vi "Queue_LV2.vi"(0 "name":string, 2 "Queue Operations":T1(ring), 5 "States[]":string[](array[string]), 7 "State":string, 11 "error in":errorcluster) -> (4 "DQ State":string, 15 "error out":errorcluster)   [LabVIEW 2020, in "Airplane CLD1.lvlib"]
uses:
  Airplane CLD1.lvlib
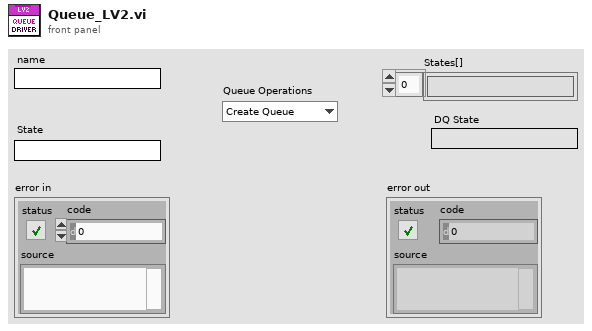
[diagram p1: front panel]
types:
  T1 = enum16{"Create Queue", "Enqueue element", "Enqueue N elements", "Dequeue", "Enstack 1 element", "Flush Queue", "Close Queue"}
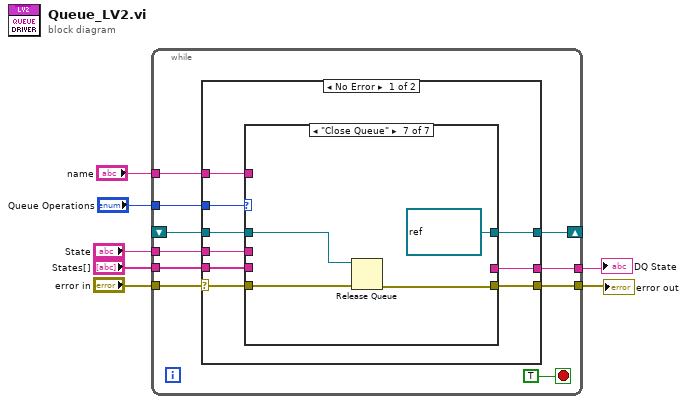
[diagram p0: block diagram]
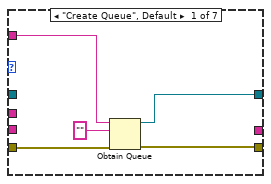
[diagram p2: hidden frame]
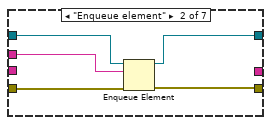
[diagram p3: hidden frame]
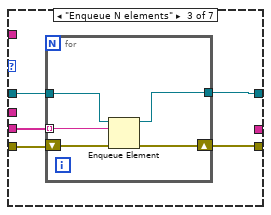
[diagram p4: hidden frame]
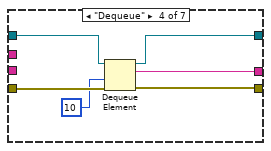
[diagram p5: hidden frame]
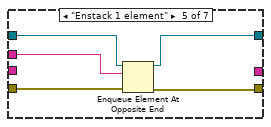
[diagram p6: hidden frame]
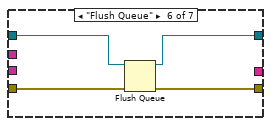
[diagram p7: hidden frame]
diagram:
  n1 = while {
    tunnel: "error in" -> [w17]
    tunnel: [w16] -> w6
    tunnel: "Queue Operations" -> [w15]
    tunnel: "name" -> [w14]
    shift-right: [w12] -> _
    shift-left: _ -> [w13]
    tunnel: "States[]" -> [w11]
    tunnel: "State" -> [w10]
    tunnel: [w9] -> w1
    stop <- TRUE stop-if-true
    n2 = case shown="No Error" w17 {
      selector: w17 -> [w26 w67]
      tunnel: [w25 w67] -> w16
      tunnel: w15 -> [w24 _]
      tunnel: w14 -> [w23 _]
      tunnel: w13 -> [w22 w66]
      tunnel: [w21 w66] -> w12
      tunnel: w11 -> [w20 _]
      tunnel: w10 -> [w19 _]
      tunnel: [w18 _] -> w9
      frame No Error {
        n3 = case shown="\"Close Queue\"" w24 {
          tunnel: [w30 w35 w40 w51 w56 w61 w64] -> w25
          tunnel: w26 -> [w31 w36 w41 w52 w57 w60 w65]
          tunnel: w23 -> [w29 _ _ _ _ _ _]
          tunnel: w22 -> [_ w34 w39 w49 w54 w59 w63]
          tunnel: [w27 w33 w38 w50 w55 w58 refnum<queue> refnum ("queue out")] -> w21
          tunnel: w20 -> [_ _ w37 _ _ _ _]
          tunnel: w19 -> [_ w32 _ _ w53 _ _]
          tunnel: [_ _ _ w47 _ _ _] -> w18
          frame "Create Queue", Default {
            n4 = Obtain Queue(name (unnamed)=w29, element data type="", error in (no error)=w31) -> (queue out=w27:refnum<queue>, error out=w30:errorcluster)  [unwired: 2 in, 1 out]
          }
          frame "Enqueue element" {
            n5 = Enqueue Element(queue=w34, element=w32, error in (no error)=w36) -> (queue out=w33:refnum<queue>, error out=w35:errorcluster)  [unwired: 1 in, 1 out]
          }
          frame "Enqueue N elements" {
            n6 = for {
              tunnel: w39 -> [w44]
              tunnel: [w43] -> w38
              shift-right: [w45] -> w40
              shift-left: w41 -> [w46]
              tunnel: w37 -> [w42] mode=indexing
              n7 = Enqueue Element(queue=w44, element=w42, error in (no error)=w46) -> (queue out=w43:refnum<queue>, error out=w45:errorcluster)  [unwired: 1 in, 1 out]
            }
          }
          frame "Dequeue" {
            n8 = Dequeue Element(queue=w49, timeout in ms (-1)=10, error in (no error)=w52) -> (queue out=w50:refnum<queue>, element=w47:string, error out=w51:errorcluster)  [unwired: 1 out]
          }
          frame "Enstack 1 element" {
            n9 = Enqueue Element At Opposite End(queue=w54, element=w53, error in (no error)=w57) -> (queue out=w55:refnum<queue>, error out=w56:errorcluster)  [unwired: 1 in, 1 out]
          }
          frame "Flush Queue" {
            n10 = Flush Queue(queue=w59, error in (no error)=w60) -> (queue out=w58:refnum<queue>, error out=w61:errorcluster)  [unwired: 1 out]
          }
          frame "Close Queue" {
            n11 = Release Queue(queue=w63, error in (no error)=w65) -> (error out=w64:errorcluster)  [unwired: 1 in, 2 out]
          }
        }
      }
      frame Error {
      }
    }
  }
  "error out" <- w6
  "DQ State" <- w1
